vi "vicon_Amatrix.vi"(0 "viconData":dbl[](array[numeric]), 1 "Constants HL":T2={"Frame Points"=[], "Brace Points in P"=[], "QP_lb"=[], "QP_ub"=[], "Q for QP"=[], "nMotors"=0, "QP stopping criteria"={"function tolerance"=1e-08, "parameter tolerance"=1000000.0, "max iterations"=10000, "max function calls"=10000, "gradient tolerance"=1000000.0, "max time (sec)"=-1.0}, "MotorsPos_wrt_Markers"=[], "nMotors 1"=0, "nMotors 2"=0, "MotorsPos_wrt_Markers pel"=[], "Frame Points_pel"=[], "Brace Points in P_pel"=[], "QP_lb pel"=[], "QP_ub pel"=[], "Q for QP pel"=[], "MotorsPos_wrt_Markers knees"=[], "nMotors 3"=0}) -> (6 "cables unit vect":T1, 7 "A Matrix":T1)   [LabVIEW 2017]
uses:
  <vilib>/Analysis/Matrix/Datatypes/RealMatrix.ctl
  typeDef/constants_HL.ctl
  <vilib>/gmath/NumericalOptimization/stopping criteria.ctl
  <vilib>/Analysis/Matrix/Numeric/Multiply/Multiply - RM,RM.vi
  <vilib>/Analysis/Matrix/Numeric/Subtract/Subtract - RM,RM.vi
  <vilib>/Analysis/7linalg.llb/Create Special Real Matrix.vi
  <vilib>/Analysis/Matrix/NI_Matrix.lvlib
  <vilib>/Analysis/NI_AALPro.lvlib
  <vilib>/gmath/NI_Gmath.lvlib
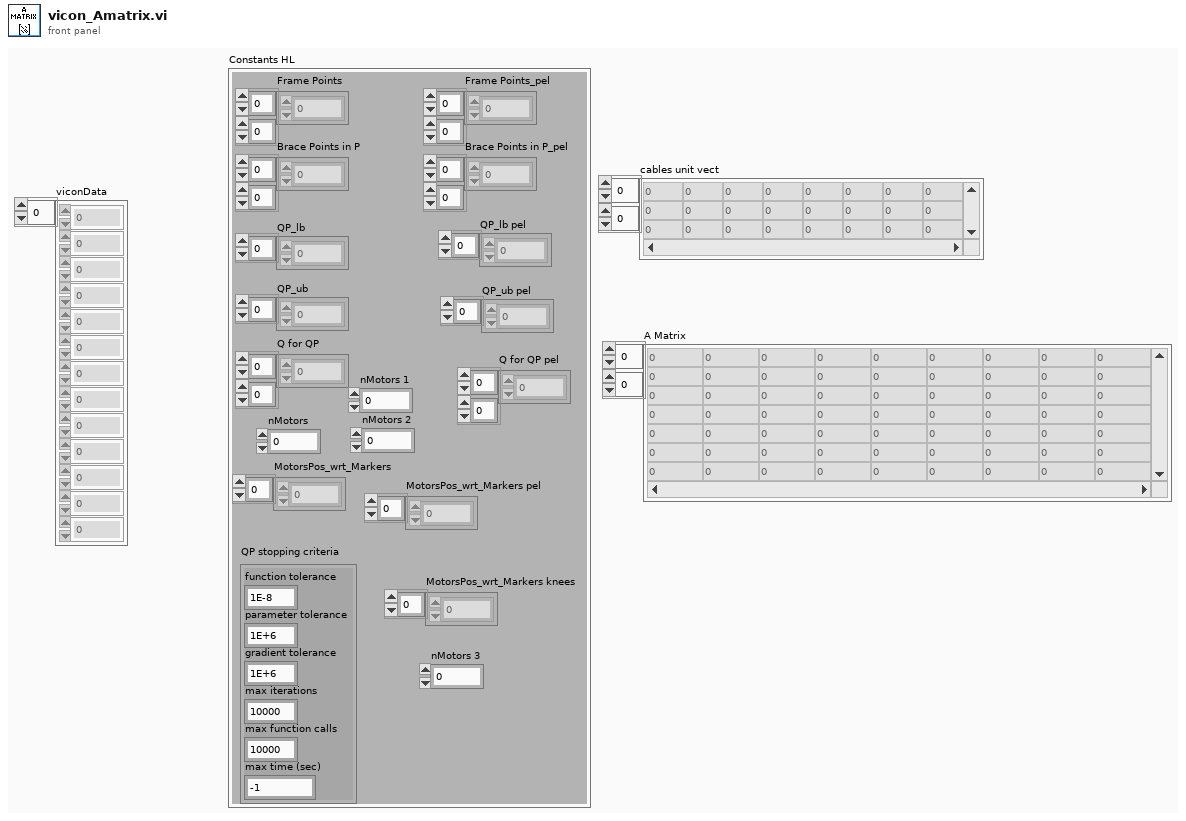
[diagram p1: front panel]
types:
  T1 = typedef "NI_Matrix.lvlib/RealMatrix.ctl" = dbl[][]
  T2 = typedef "constants_HL.ctl" = cluster{"Frame Points":dbl[][], "Brace Points in P":dbl[][], "QP_lb":dbl[], "QP_ub":dbl[], "Q for QP":dbl[][], "nMotors":i32, "QP stopping criteria":T3, "MotorsPos_wrt_Markers":i32[], "nMotors 1":i32, "nMotors 2":i32, "MotorsPos_wrt_Markers pel":i32[], "Frame Points_pel":dbl[][], "Brace Points in P_pel":dbl[][], "QP_lb pel":dbl[], "QP_ub pel":dbl[], "Q for QP pel":dbl[][], "MotorsPos_wrt_Markers knees":i32[], "nMotors 3":i32}
  T3 = typedef "NI_Gmath.lvlib/stopping criteria.ctl" = cluster{"function tolerance":dbl, "parameter tolerance":dbl, "max iterations":i32, "max function calls":i32, "gradient tolerance":dbl, "max time (sec)":dbl}
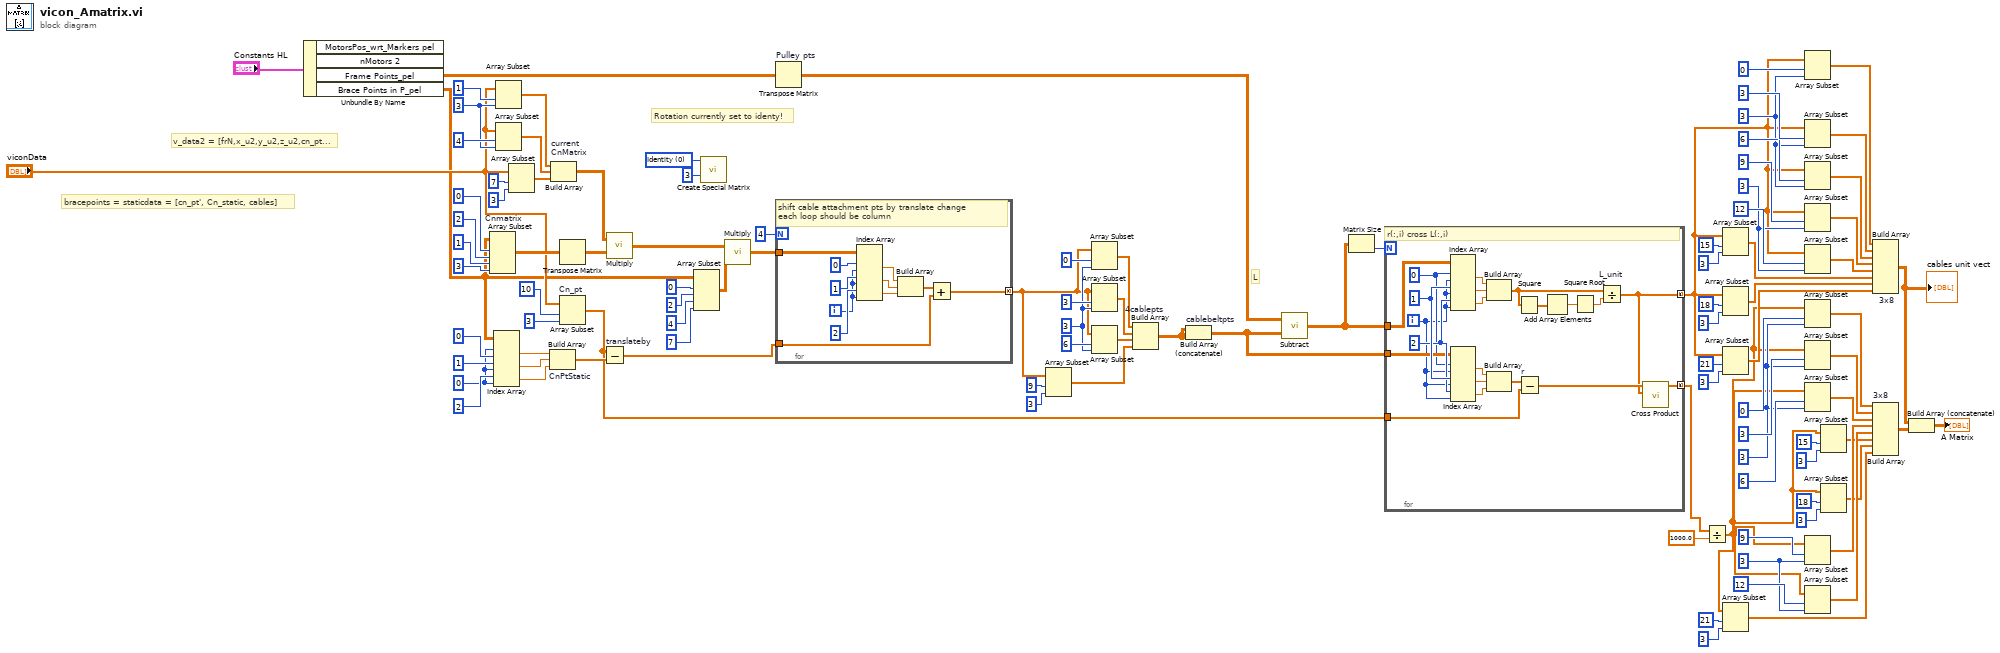
[diagram p0: block diagram]
diagram:
  w3 = 0 items=["Identity", "Diagonal", "Toeplitz", "Vandermonde", "Companion", "Hankel", "Hadamard", "Wilkinson", "Hilbert", "Inverse Hilbert", "Rosser", "Pascal"] ("matrix type")
  w23 = 3 ("length")
  w30 = 3 ("length")
  w45 = 3 ("length")
  w52 = 3 ("length")
  w64 = 3 ("length")
  w93 = 3 ("length")
  w101 = 0 ("index (row)")
  # "Rotation currently set to identy!"
  # "L"
  # "v_data2 = [frN,x_u2,y_u2,z_u2,cn_pt..."
  # "bracepoints = staticdata = [cn_pt', Cn_static, cables]"
  n1 = Unbundle By Name("Constants HL") -> ("Frame Points_pel"=w7:dbl[][], "Brace Points in P_pel"=w8:dbl[][])  [unwired: 2 out]
  n2 = Array Subset "Cnmatrix"(array=w8, index (row)=0 ("row 1"), length (row)=2 ("row N"), index (col)=1 ("column 1"), length (col)=3 ("column N")) -> (w84:dbl[][])
  n3 = Index Array(array=w8, index (row) #1=w101, index (col) #1=0 ("index (col)"), index (row) #2=1 ("index (row)"), index (col) #2=w101, index (row) #3=2 ("index (row)"), index (col) #3=w101) -> (element #1=w100:dbl, element #2=w99:dbl, element #3=w98:dbl)
  n4 = Array Subset(array="viconData", index=1, length=w93) -> (w95:dbl[])
  n5 = Array Subset(array="viconData", index=4, length=w93) -> (w92:dbl[])
  n6 = Array Subset(array="viconData", index=7, length=3) -> (w89:dbl[])
  n7 = Build Array "CnPtStatic"(w100, w99, w98) -> (w97:dbl[])
  n8 = Build Array "current\nCnMatrix"(w95, w92, w89) -> (w82:T1)
  n9 = Array Subset "Cn_pt"(array="viconData", index=10, length=3) -> (w73:dbl[])
  n10 = Transpose Matrix(1:w84) -> (0:w83:dbl[][])
  n11 = Subtract "translateby"(x=w73, y=w97) -> (x-y=w76:dbl[])
  n12 = call-poly <vilib>:"Multiply.vi"("Real Matrix B"=w83, "Real Matrix A"=w82) -> ("A * B"=w1:T1)
  n13 = Array Subset(array=w8, index (row)=0 ("row 1"), length (row)=2 ("row N"), index (col)=4 ("column 1"), length (col)=7 ("column N")) -> (w77:dbl[][])
  n14 = call-poly <vilib>:"Create Special Matrix.vi"("matrix type"=w3, "matrix size"=3) -> ()  [unwired: 3 in, 2 out]
  n15 = call-poly <vilib>:"Multiply.vi"("Real Matrix B"=w77, "Real Matrix A"=w1) -> ("A * B"=w72:T1)
  n16 = Transpose Matrix "Pulley pts"(1:w7) -> (0:w75:dbl[][])
  n17 = for {
    N: 4 -> [_]
    tunnel: w76 -> [w117]
    tunnel: [w116] -> w57 mode=concatenating
    tunnel: w72 -> [w115]
    i -> [w111]
    # "shift cable attachment pts by translate change\neach loop should be column"
    n18 = Index Array(array=w115, index (row) #1=0 ("index (row)"), index (col) #1=w111, index (row) #2=1 ("index (row)"), index (col) #2=w111, index (row) #3=2 ("index (row)"), index (col) #3=w111) -> (element #1=w110:dbl, element #2=w109:dbl, element #3=w108:dbl)
    n19 = Build Array(w110, w109, w108) -> (w107:dbl[])
    n20 = Add ("Add.vi")(x=w107, y=w117) -> (x+y=w116:dbl[])
  }
  n21 = Array Subset(array=w57, index=9, length=3) -> (w58:dbl[])
  n22 = Array Subset(array=w57, index=0, length=w64) -> (w63:dbl[])
  n23 = Array Subset(array=w57, index=3, length=w64) -> (w60:dbl[])
  n24 = Array Subset(array=w57, index=6, length=w64) -> (w59:dbl[])
  n25 = Build Array "4cablepts"(w63, w60, w59, w58) -> (w56:T1)
  n26 = Build Array (concatenate) "cablebeltpts"(w56, w56) -> (w74:T1)
  n27 = call-poly <vilib>:"Subtract.vi"("Real Matrix B"=w74, "Real Matrix A"=w75) -> ("A - B"=w69:T1)
  n28 = Matrix Size(0:w69) -> (2:w68:i32)  [unwired: 1 out]
  n29 = for {
    N: w68 -> [_]
    tunnel: w74 -> [w121]
    tunnel: w73 -> [w138]
    tunnel: w69 -> [w136]
    tunnel: [w132] -> w4 mode=concatenating
    tunnel: [w118] -> w12 mode=concatenating
    i -> [w119]
    w127 = 2 ("index (row)")
    w128 = 1 ("index (row)")
    w120 = 0 ("index (row)")
    # "r(:,i) cross L(:,i)"
    n30 = Index Array(array=w136, index (row) #1=w120, index (col) #1=w119, index (row) #2=w128, index (col) #2=w119, index (row) #3=w127, index (col) #3=w119) -> (element #1=w135:dbl, element #2=w134:dbl, element #3=w133:dbl)
    n31 = Index Array(array=w121, index (row) #1=w120, index (col) #1=w119, index (row) #2=w128, index (col) #2=w119, index (row) #3=w127, index (col) #3=w119) -> (element #1=w131:dbl, element #2=w130:dbl, element #3=w129:dbl)
    n32 = Build Array(w135, w134, w133) -> (w122:dbl[])
    n33 = Build Array(w131, w130, w129) -> (w126:dbl[])
    n34 = Square(x=w122) -> (x^2=w124:dbl[])
    n35 = Subtract "r"(x=w126, y=w138) -> (x-y=w137:dbl[])
    n36 = Add Array Elements(numeric array=w124) -> (sum=w125:dbl)
    n37 = Square Root(x=w125) -> (sqrt(x)=w123:dbl)
    n38 = Divide "L_unit"(x=w122, y=w123) -> (x/y=w118:dbl[])
    n39 = call <vilib>:"Cross Product.vi"("B Vector"=w118, "A Vector"=w137) -> ("Cross Product"=w132:dbl[])  [unwired: 8 in, 1 out]
  }
  n40 = Divide(x=w4, y=1000.0) -> (x/y=w5:dbl[])
  n41 = Array Subset(array=w12, index=15, length=3) -> (w19:dbl[])
  n42 = Array Subset(array=w12, index=18, length=3) -> (w16:dbl[])
  n43 = Array Subset(array=w12, index=21, length=3) -> (w13:dbl[])
  n44 = Array Subset(array=w5, index=21, length=3) -> (w35:dbl[])
  n45 = Array Subset(array=w12, index=0, length=w30) -> (w29:dbl[])
  n46 = Array Subset(array=w12, index=3, length=w30) -> (w27:dbl[])
  n47 = Array Subset(array=w12, index=6, length=w30) -> (w26:dbl[])
  n48 = Array Subset(array=w12, index=9, length=w23) -> (w25:dbl[])
  n49 = Array Subset(array=w12, index=12, length=w23) -> (w20:dbl[])
  n50 = Array Subset(array=w5, index=0, length=w52) -> (w51:dbl[])
  n51 = Array Subset(array=w5, index=3, length=w52) -> (w49:dbl[])
  n52 = Array Subset(array=w5, index=6, length=w52) -> (w48:dbl[])
  n53 = Array Subset(array=w5, index=9, length=w45) -> (w47:dbl[])
  n54 = Array Subset(array=w5, index=12, length=w45) -> (w42:dbl[])
  n55 = Array Subset(array=w5, index=15, length=3) -> (w41:dbl[])
  n56 = Array Subset(array=w5, index=18, length=3) -> (w38:dbl[])
  n57 = Build Array "3x8"(w29, w27, w26, w25, w20, w19, w16, w13) -> (w11:T1)
  "cables unit vect" <- w11
  n58 = Build Array "3x8"(w51, w49, w48, w47, w42, w41, w38, w35) -> (w34:T1)
  n59 = Build Array (concatenate)(w11, w34) -> (→"A Matrix":T1)
